vi "DifferentStdPrototype.vi"(2 "Invocation info":T1, 3 "Input buffer":T4, 4 "Sequence Context":T2) -> (0 "error out":errorcluster, 1 "Test Data":T3 {"Numeric Measurement" format="%.2f"})   [LabVIEW 2010]
uses:
  LabVIEW Test - Input Buffer.ctl
  LabVIEW Test - Test Data.ctl
  LabVIEW Test - Sequence Context.ctl
  LabVIEW Test - Invocation Info.ctl
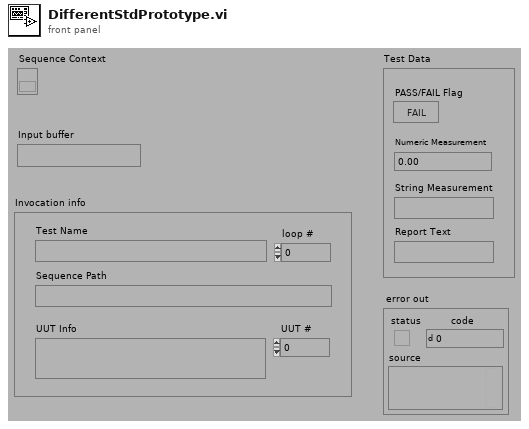
[diagram p1: front panel]
types:
  T1 = typedef "LabVIEW Test - Invocation Info.ctl" = cluster{"UUT #":i32, "loop #":i32, "UUT Info":string, "Test Name":string, "Sequence Path":string}
  T2 = typedef "LabVIEW Test - Sequence Context.ctl" = refnum<k7>
  T3 = typedef "LabVIEW Test - Test Data.ctl" = cluster{"PASS/FAIL Flag":bool, "Numeric Measurement":dbl, "String Measurement":string, "Report Text":string}
  T4 = typedef "LabVIEW Test - Input Buffer.ctl" = string
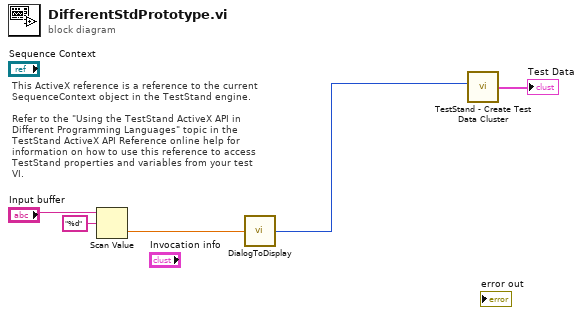
[diagram p0: block diagram]
diagram:
  # "This ActiveX reference is a reference to the current\nSequenceContext object in the TestStand engine.\n\nRefer to the \"Using the TestStand ActiveX API in\nDifferent Programming Languages\" topic in the \nTestStand ActiveX API Reference online help for\ninformation on how to use this reference to access\nTestStand properties and variables from your test VI."
  n1 = Scan Value(string="Input buffer", format string="%d") -> (value=w2:dbl)  [unwired: 2 out]
  n2 = call "DialogToDisplay.vi"("Numeric"=w2) -> ("Numeric 2"=w1:i32)
  n3 = call "TestStand - Create Test Data Cluster.vi"("Numeric Measurement"=w1) -> ("Test Data"=→"Test Data":T3)  [unwired: 3 in]
